vi "waveform_numeric.vi"() -> ()   [LabVIEW 2019]
uses:
  <instrlib>/Yokogawa PZ4000/Yokogawa PZ4000.lvlib
  <vilib>/Utility/file.llb/Write Delimited Spreadsheet (DBL).vi
panel:
  out "numeric":T1
  in  "dt integracao":dbl=1.0 format="%#_13g"
  out "waveform cluster":T1
  out "waveforms":dbl[][](graph)
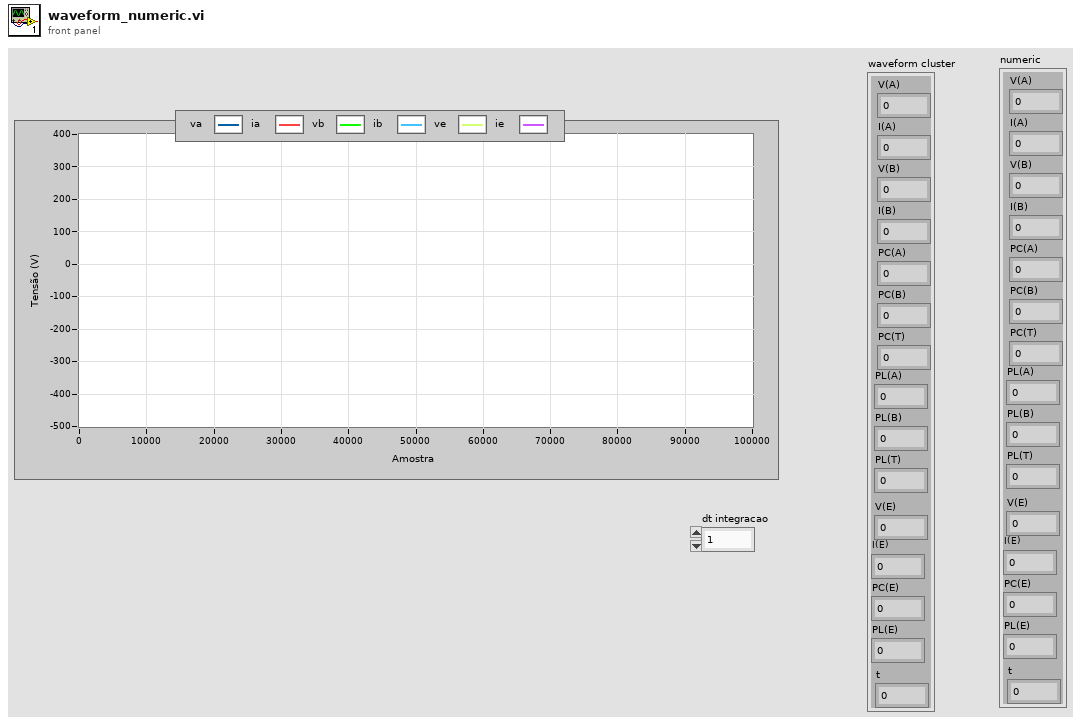
[diagram p1: front panel]
types:
  T1 = cluster{"V(A)":dbl, "I(A)":dbl, "V(B)":dbl, "I(B)":dbl, "PC(A)":dbl, "PC(B)":dbl, "PC(T)":dbl, "PL(T)":dbl, "PL(B)":dbl, "PL(A)":dbl, "V(E)":dbl, "PL(E)":dbl, "PC(E)":dbl, "I(E)":dbl, "t":dbl}
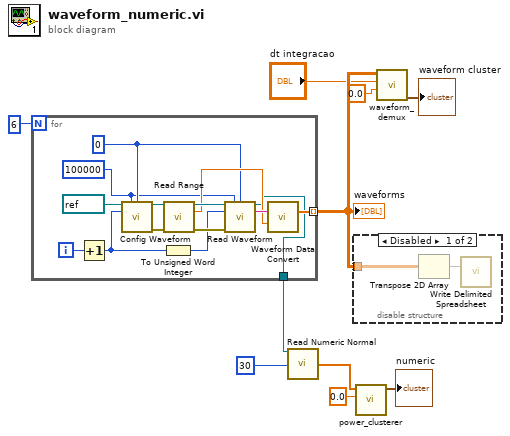
[diagram p0: block diagram]
diagram:
  n1 = for {
    N: 6 -> [_]
    tunnel: [w12] -> w9 mode=indexing
    tunnel: [w11] -> w5
    i -> [w14]
    w17 = u32 0 ("Start Point (0)")
    w16 = u32 100000 ("End Point (1000)")
    n2 = Increment(x=w14) -> (x+1=w13:i32)
    n3 = call <instrlib>:"Config Waveform.vi"("VISA resource name"=refnum<visa-resource-name> "PZ", "End Point (1000)"=w16, "Start Point (0)"=w17, "Select Trace (1)"=w13) -> ("VISA resource name out"=w19:refnum<visa-resource-name>, "error out"=w18:errorcluster)  [unwired: 10 in]
    n4 = To Unsigned Word Integer(number=w13) -> (unsigned 16bit integer=w20:u16)
    n5 = call <instrlib>:"Read Range.vi"("VISA resource name"=w19, "error in (no error)"=w18) -> ("VISA resource name out"=w24:refnum<visa-resource-name>, "Range"=w21:dbl, "error out"=w23:errorcluster)  [unwired: 11 in]
    n6 = call <instrlib>:"Read Waveform.vi"("VISA resource name"=w24, "End Point (1000)"=w16, "Start Point (0)"=w17, "Select Trace (1)"=w20, "error in (no error)"=w23) -> ("VISA resource name out"=w11:refnum<visa-resource-name>, "Waveform Data"=w22:string)  [unwired: 8 in, 1 out]
    n7 = call <instrlib>:"Waveform Data Convert.vi"("Input Data"=w22, "Range"=w21) -> ("Output"=w12:dbl[])  [unwired: 11 in, 2 out]
  }
  "waveforms" <- w9
  n8 = call <instrlib>:"Read Numeric Normal.vi"("VISA resource name"=w5, "Number of Item (15)"=u16 30) -> ("Measure"=w3:dbl[])  [unwired: 10 in, 3 out]
  n9 = disable-structure shown="Disabled" {
    disable-tunnel: w9 -> [w26 _]
    frame Disabled {
      n10 = Transpose 2D Array(2D array=w26) -> (transposed array=w25:dbl[][])
      n11 = call-poly <vilib>:"Write Delimited Spreadsheet.vi"("2D data"=w25) -> ()  [unwired: 13 in, 2 out]
    }
    frame Enabled {
    }
  }
  n12 = call "power_clusterer.vi"("relative seconds"=0.0, "Measure"=w3) -> ("Cluster"=→"numeric":T1)  [unwired: 9 in]
  n13 = call "waveform_demux.vi"("t"=0.0, "dt integracao"="dt integracao", "Output"=w9) -> ("watt num cluster"=→"waveform cluster":T1)  [unwired: 5 in, 3 out]
